vi "13RomanToInteger.vi"(8 "error in (no error)":errorcluster, 11 "String":string) -> (0 "error out":errorcluster, 3 "Numeric":i32)   [LabVIEW 2023]
panel:
  out "Array 2":i32[](array[numeric])
  out "Array":string[](array[string])
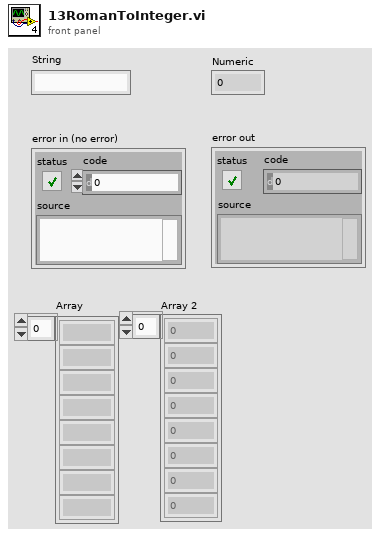
[diagram p1: front panel]
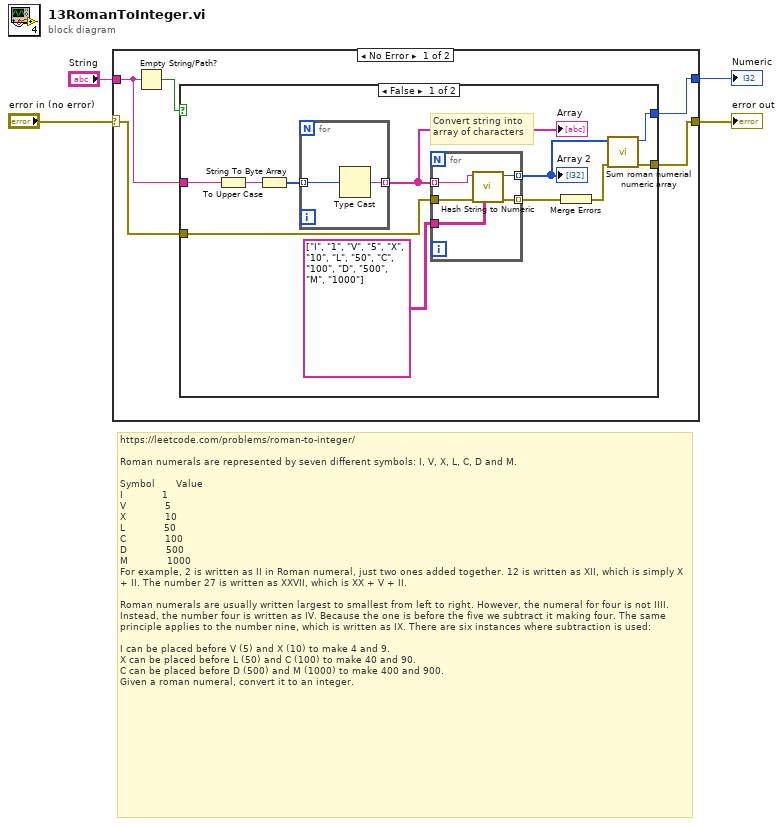
[diagram p0: block diagram]
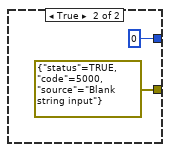
[diagram p2: hidden frame]
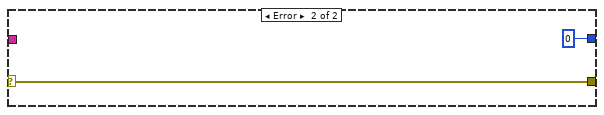
[diagram p3: hidden frame]
diagram:
  # "https://leetcode.com/problems/roman-to-integer/\n\nRoman numerals are represented by seven different symbols: I, V, X, L, C, D and M.\n\nSymbol       Value\nI             1\nV             5\nX             10\nL             50\nC             100\nD             500\nM             1000\nFor example, 2 is written as II in Roman numeral, just two ones added together. 12 is written as XII, which is simply X + II. The number 27 is written as XXVII, which is XX + V + II.\n\nRoman numerals are usually written largest to smallest from left to right. However, the numeral for four is not IIII. Instead, the number four is written as IV. Because the one is before the five we subtract it making four. The same principle applies to the number nine, which is written as IX. There are six instances where subtraction is used:\n\nI can be placed before V (5) and X (10) to make 4 and 9. \nX can be placed before L (50) and C (100) to make 40 and 90. \nC can be placed before D (500) and M (1000) to make 400 and 900.\nGiven a roman numeral, convert it to an integer."
  n1 = case shown="No Error" "error in (no error)" {
    selector: "error in (no error)" -> [w9 w31]
    tunnel: "String" -> [w6 _]
    tunnel: [w8 w31] -> w2
    tunnel: [w7 0] -> w1
    frame No Error {
      n2 = Empty String/Path?(string/path=w6) -> (empty?=w5:bool)
      n3 = case shown="False" w5 {
        tunnel: w9 -> [w17 _]
        tunnel: [w10 errorcluster {"status"=TRUE, "code"=5000, "source"="Blank string input"} ("error IO")] -> w8
        tunnel: [w12 0] -> w7
        tunnel: w6 -> [w14 _]
        frame False {
          # "Convert string into\narray of characters"
          n4 = To Upper Case(1:w14) -> (0:w15:string)
          n5 = String To Byte Array(string=w15) -> (unsigned byte array=w20:u8[])
          n6 = for {
            tunnel: w20 -> [w27] mode=indexing
            tunnel: [w26] -> w18 mode=indexing
            n7 = Type Cast(x=w27) -> (*(type *) &x=w26:string)  [unwired: 1 in]
          }
          "Array" <- w18
          n8 = for {
            tunnel: string[][] [["I", "1"], ["V", "5"], ["X", "10"], ["L", "50"], ["C", "100"], ["D", "500"], ["M", "1000"]] -> [w25]
            tunnel: w18 -> [w24] mode=indexing
            tunnel: [w23] -> w13 mode=indexing
            tunnel: w17 -> [w22]
            tunnel: [w21] -> w16 mode=indexing
            n9 = call "Hash String to Numeric.vi"("Hash Array"=w25, "error in (no error)"=w22, "String Input"=w24) -> ("error out"=w21:errorcluster, "Numeric Output"=w23:i32)  [unwired: 7 in]
          }
          "Array 2" <- w13
          n10 = Merge Errors(w16) -> (w11:errorcluster)
          n11 = call "Sum roman numerial numeric array.vi"("error in (no error)"=w11, "Roman numeral array"=w13) -> ("error out"=w10:errorcluster, "Summed array"=w12:i32)  [unwired: 8 in]
        }
        frame True {
        }
      }
    }
    frame Error {
    }
  }
  "Numeric" <- w1
  "error out" <- w2
